vi "ROVFifoClosePing.vi"(11 "Cluster in":T1={"Connections"={"Ping1D - A"={"Connection"="", "error"={"status"=FALSE, "code"=0, "source"=""}, "Distance"=0.0, "FIFO"={"rt fifo"=refnum, "error"={"status"=FALSE, "code"=0, "source"=""}}}, "Ping1D - B"={"Connection"="", "error"={"status"=FALSE, "code"=0, "source"=""}, "Distance"=0.0, "FIFO"={"rt fifo"=refnum, "error"={"status"=FALSE, "code"=0, "source"=""}}}, "IMU"={"Error"={"status"=FALSE, "code"=0, "source"=""}, "FIFO"={"fifo"=refnum, "error"={"status"=FALSE, "code"=0, "source"=""}}}, "MotorControl"={"Rear"={"Error PWM"={"status"=FALSE, "code"=0, "source"=""}, "Error Direction"={"status"=FALSE, "code"=0, "source"=""}}, "Left"={"Error PWM"={"status"=FALSE, "code"=0, "source"=""}, "Error Direction"={"status"=FALSE, "code"=0, "source"=""}}, "Right"={"Error PWM"={"status"=FALSE, "code"=0, "source"=""}, "Error Direction"={"status"=FALSE, "code"=0, "source"=""}}}}, "sensorData"={"IMU Data"={"X-Axis"=0.0, "Y-Axis"=0.0, "Z-Axis"=0.0}}, "outputData"={"Rotation Angle"=0.0, "Rotation Vector"={"x"=0.0, "y"=0.0, "z"=0.0}, "PING A distance"=0.0, "Ping B distance"=0.0, "angles"={"roll"=0.0, "pitch"=0.0, "yaw"=0.0}}, "Writer"={"endpoint"="", "error"={"status"=FALSE, "code"=0, "source"=""}}, "PID"={"reinitialize?"=FALSE, "Depth"={"setpoint"=0.0, "Gains"={"proportional gain (Kc)"=1.0, "integral time (Ti, min)"=0.01, "derivative time (Td, min)"=0.0}}, "Roll"={"setpoint"=0.0, "Gains"={"proportional gain (Kc)"=1.0, "integral time (Ti, min)"=0.01, "derivative time (Td, min)"=0.0}}}} {"PID"."Roll"."setpoint" format="%.2f"; "PID"."Roll"."Gains"."derivative time (Td, min)" format="%.3f"; "PID"."Roll"."Gains"."integral time (Ti, min)" format="%.3f"; "PID"."Roll"."Gains"."proportional gain (Kc)" format="%.3f"; "PID"."Depth"."setpoint" format="%.2f"; "PID"."Depth"."Gains"."derivative time (Td, min)" format="%.3f"; "PID"."Depth"."Gains"."integral time (Ti, min)" format="%.3f"; "PID"."Depth"."Gains"."proportional gain (Kc)" format="%.3f"}) -> (0 "error Ping B Fifo":errorcluster, 1 "error Ping A Fifo":errorcluster)   [LabVIEW 2019]
uses:
  Connections.ctl
  ROVsensorData.ctl
  ROVdataOut.ctl
  ROVcluster.ctl
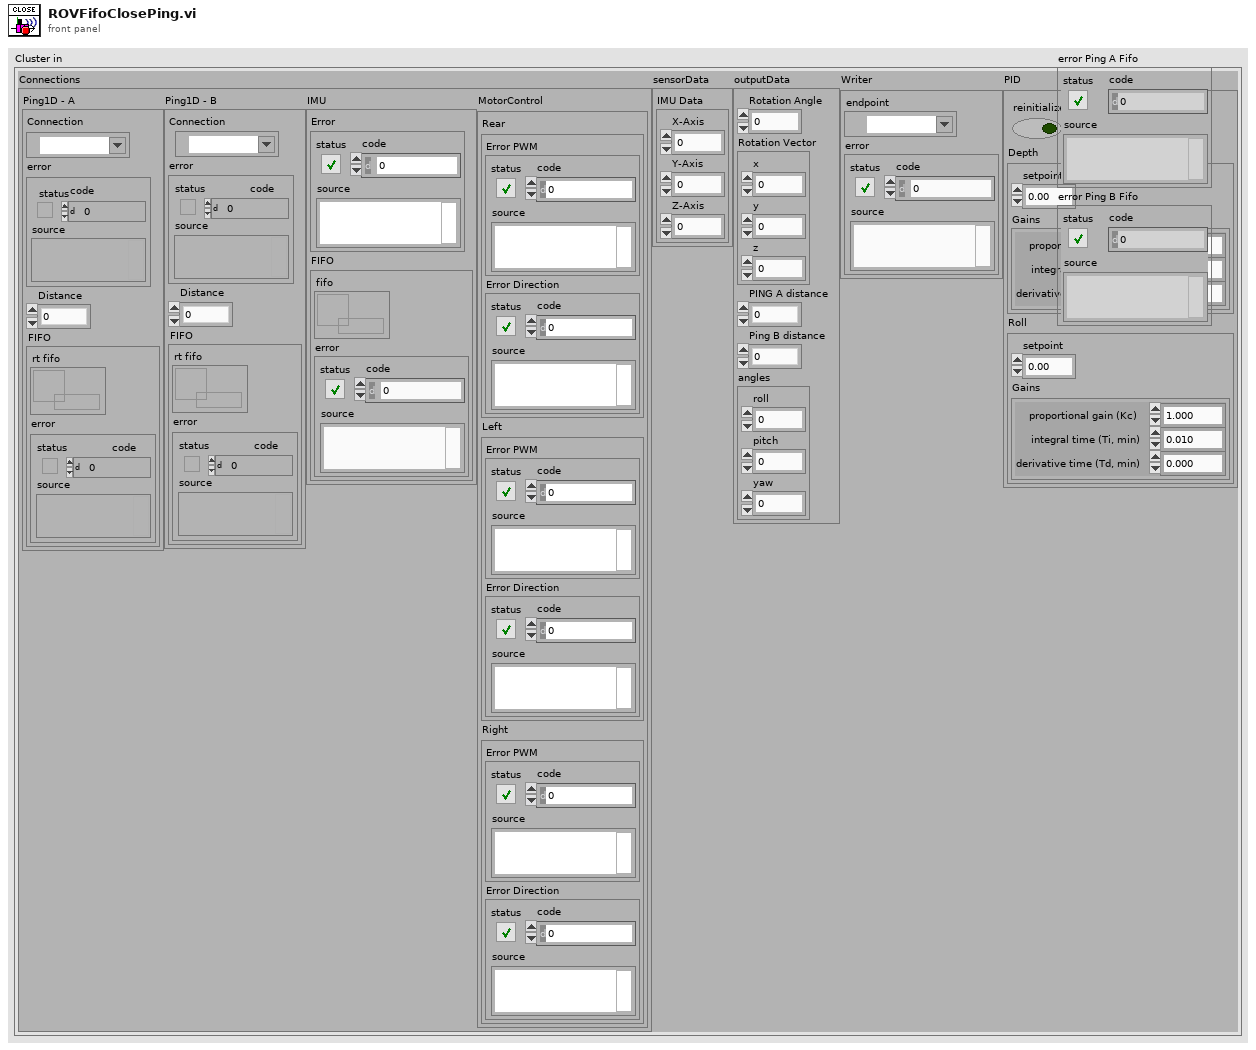
[diagram p1: front panel]
types:
  T1 = typedef "ROVcluster.ctl" = cluster{"Connections":T2, "sensorData":T3, "outputData":T4, "Writer":cluster{"endpoint":refnum<k21>, "error":errorcluster}, "PID":cluster{"reinitialize?":bool, "Depth":cluster{"setpoint":dbl, "Gains":cluster{"proportional gain (Kc)":dbl, "integral time (Ti, min)":dbl, "derivative time (Td, min)":dbl}}, "Roll":cluster{"setpoint":dbl, "Gains":cluster{"proportional gain (Kc)":dbl, "integral time (Ti, min)":dbl, "derivative time (Td, min)":dbl}}}}
  T2 = typedef "Connections.ctl" = cluster{"Ping1D - A":cluster{"Connection":refnum<visa-resource-name>, "error":errorcluster, "Distance":dbl, "FIFO":cluster{"rt fifo":refnum<k33>, "error":errorcluster}}, "Ping1D - B":cluster{"Connection":refnum<visa-resource-name>, "error":errorcluster, "Distance":dbl, "FIFO":cluster{"rt fifo":refnum<k33>, "error":errorcluster}}, "IMU":cluster{"Error":errorcluster, "FIFO":cluster{"fifo":refnum<k33>, "error":errorcluster}}, "MotorControl":cluster{"Rear":cluster{"Error PWM":errorcluster, "Error Direction":errorcluster}, "Left":cluster{"Error PWM":errorcluster, "Error Direction":errorcluster}, "Right":cluster{"Error PWM":errorcluster, "Error Direction":errorcluster}}}
  T3 = typedef "ROVsensorData.ctl" = cluster{"IMU Data":cluster{"X-Axis":dbl, "Y-Axis":dbl, "Z-Axis":dbl}}
  T4 = typedef "ROVdataOut.ctl" = cluster{"Rotation Angle":dbl, "Rotation Vector":cluster{"x":dbl, "y":dbl, "z":dbl}, "PING A distance":dbl, "Ping B distance":dbl, "angles":cluster{"roll":dbl, "pitch":dbl, "yaw":dbl}}
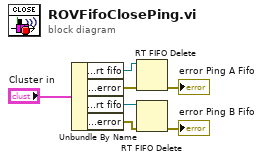
[diagram p0: block diagram]
diagram:
  n1 = Unbundle By Name("Cluster in") -> ("Connections.Ping1D - A.FIFO.rt fifo"=w6:refnum<k33>, "Connections.Ping1D - A.FIFO.error"=w5:errorcluster, "Connections.Ping1D - B.FIFO.rt fifo"=w3:refnum<k33>, "Connections.Ping1D - B.FIFO.error"=w2:errorcluster)
  n2 = RT FIFO Delete(0:w6, 3:w5) -> (11:→"error Ping A Fifo":errorcluster)  [unwired: 1 in]
  n3 = RT FIFO Delete(0:w3, 3:w2) -> (11:→"error Ping B Fifo":errorcluster)  [unwired: 1 in]
